vi "Accelerometer Alarm.vi"() -> ()   [LabVIEW 2025]
doc: "Accelerometer Example\n\nThis example shows the basic usage of an accelerometer. It will obtain a voltage value, chart it over time, and check it against bounds that are supplied by the user.\n\nThis example expects a USB cable connected from your development PC to the Type B USB Jack (next to the power input) on the roboRIO."
uses:
  <vilib>/Rock Robotics/WPI/Accelerometer/WPI_AccelerometerAnalogChannels.ctl
  <vilib>/Rock Robotics/SystemInterfaces/AI/FPGA_AIChannel.ctl
  <vilib>/Rock Robotics/WPI/Accelerometer/WPI_AccelerometerScaling.ctl
  <vilib>/Rock Robotics/WPI/Accelerometer/WPI_AccelerometerAnalogOpen.vi
panel:
  in  "Scaling":T1={"Gain (VoltsPerG)"=1.0, "Center Voltage"=2.5}
  in  "Analog Channels":T2={"X-Axis"=enum."AI 0", "Y-Axis"=enum."Invalid", "Z-Axis"=enum."Invalid"}
  out "Alarm":bool
  in  "Lower Alarm Bound":dbl=-1.0
  in  "Upper Alarm Bound":dbl=1.0
  out "Accelerometer Chart":T4(graph)
  out "Acc Value":dbl
  in  "stop":bool
  # "Set these inputs before running."
  # "These can be set while running."
  # "This chart shows the value of the accelerometer over time.  The alarm Boolean will light up when the accelerometer value is out of bounds."
  # "X"
  # "This shows wiring for an analog accelerometer."
  # "5"
  # "G"
  # "accelerometer pins"
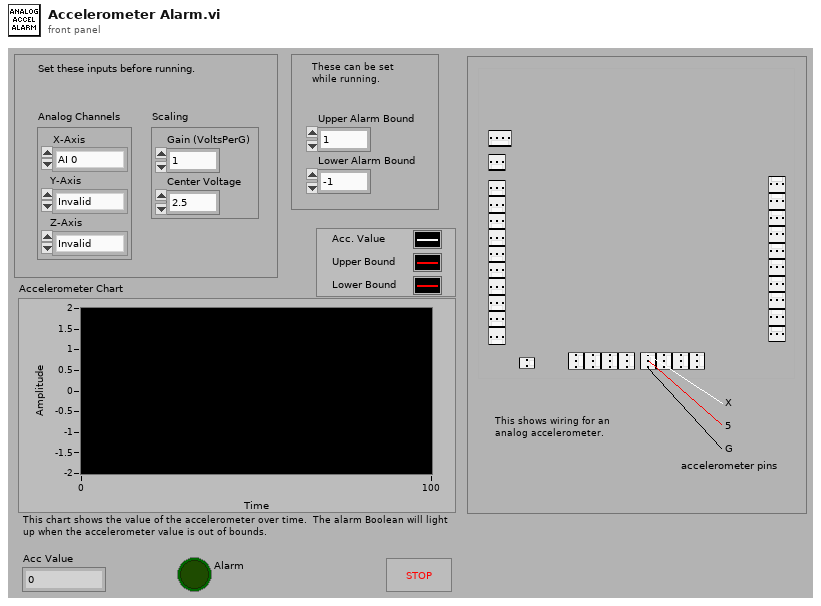
[diagram p1: front panel]
types:
  T1 = typedef "WPI_AccelerometerScaling.ctl" = cluster{"Gain (VoltsPerG)":dbl, "Center Voltage":dbl}
  T2 = typedef "WPI_AccelerometerAnalogChannels.ctl" = cluster{"X-Axis":T3, "Y-Axis":T3, "Z-Axis":T3}
  T3 = typedef "FPGA_AIChannel.ctl" = enum8{"AI 0", "AI 1", "AI 2", "AI 3", "AI MXP 0", "AI MXP 1", "AI MXP 2", "AI MXP 3", "Invalid"}
  T4 = cluster{"Acceleration":dbl, "Upper Alarm Bound":dbl, "Lower Alarm Bound":dbl}
  T5 = typedef "WPI_AccelerometerDevRef.ctl" = cluster{"DevStatus":errorcluster, "Scaling":T1, "Analog Channels":T2, "I2C Bus":T6, "SPI Bus":T7, "Accel Range":T8, "ADXL Axes":T9, "Handle":i32, "Device Address":u8, "Accel Type":enum16{"Analog", "ADXL345 I2C", "ADXL345 SPI", "Internal", "ADXL362 SPI"}}
  T6 = typedef "i2c_bus.ctl" = enum16{"I2C On-Board", "I2C MXP", "Invalid"}
  T7 = typedef "spi_bus.ctl" = enum16{"SPI On-Board, CS0", "SPI On-Board, CS1", "SPI On-Board, CS2", "SPI On-Board, CS3", "SPI MXP", "Invalid"}
  T8 = typedef "ADXL345 Range.ctl" = u8
  T9 = typedef "WPI_AccelerometerADXL345 Axes.ctl" = cluster{"X-Axis":bool, "Y-Axis":bool, "Z-Axis":bool}
  T10 = cluster{"X-Axis":dbl, "Y-Axis":dbl, "Z-Axis":dbl}
  T11 = cluster{"X-Axis":dbl, "Upper Alarm Bound":dbl, "Lower Alarm Bound":dbl}
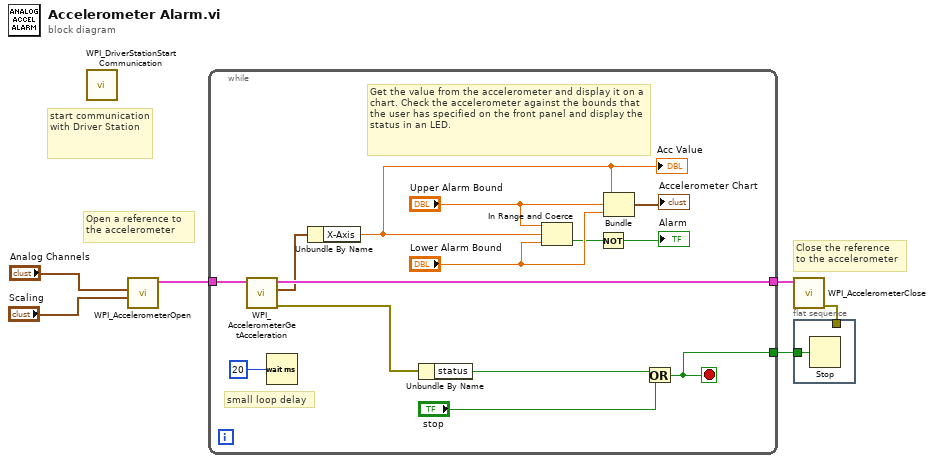
[diagram p0: block diagram]
diagram:
  # "start communication with Driver Station"
  # "Close the reference\nto the accelerometer"
  # "Open a reference to \nthe accelerometer"
  n1 = call <vilib>:"WPI_DriverStationStart Communication.vi"() -> ()  [unwired: 3 in, 9 out]
  n2 = call-poly <vilib>:"WPI_AccelerometerOpen.vi"("Scaling"="Scaling", "Analog Channels"="Analog Channels") -> ("AccelerometerDevRef"=w6:T5)  [unwired: 8 in, 1 out]
  n3 = while {
    tunnel: w6 -> [w8]
    tunnel: [w13] -> w4
    tunnel: [w18] -> w5
    stop <- w13 stop-if-true
    # "small loop delay"
    # "Get the value from the accelerometer and display it on a chart. Check the accelerometer against the bounds that the user has specified on the front panel and display the status in an LED."
    n4 = call <vilib>:"WPI_AccelerometerGetAcceleration.vi"("AccelerometerDevRef"=w8) -> ("error out"=w11:errorcluster, "Accelerations"=w10:T10, "AccelerometerDevRef"=w18:T5)  [unwired: 1 in, 7 out]
    n5 = Wait (ms)(milliseconds to wait=u32 20) -> ()  [unwired: 1 out]
    n6 = Unbundle By Name(w10) -> ("X-Axis"=w7:dbl)
    "Acc Value" <- w7
    n7 = Unbundle By Name(w11) -> ("status"=w14:bool)
    n8 = In Range and Coerce(upper limit="Upper Alarm Bound", x=w7, lower limit="Lower Alarm Bound") -> (In Range?=w15:bool)  [unwired: 1 out]
    n9 = Not(x=w15) -> (.not. x?=→"Alarm":bool)
    n10 = Bundle("X-Axis"=w7, "Upper Alarm Bound"="Upper Alarm Bound", "Lower Alarm Bound"="Lower Alarm Bound") -> (→"Accelerometer Chart":T11)  [unwired: 1 out]
    n11 = Or(x=w14, y="stop") -> (x .or. y?=w13:bool)
  }
  n12 = call <vilib>:"WPI_AccelerometerClose.vi"("AccelerometerDevRef"=w5) -> ("error out"=w3:errorcluster)  [unwired: 1 in, 9 out]
  n13 = flat-sequence {
    tunnel: w4 -> [w21]
    tunnel: w3 -> [_]
    frame #0 {
      n14 = Stop(stop? (T)=w21) -> ()
    }
  }
